vi "getMultiBarCode.vi"() -> ()   [LabVIEW 2012]
uses:
  <vilib>/vision/NI_Vision_Development_Module.lvlib
panel:
  out "String 4":string
  out "String 3":string
  out "String 2":string
  out "String":string
  in  "Stop":bool
  in  "Delay (s.)":dbl(slide)=0.4897959183673469 scale=0.0..2.0
  out "Code Read":string
  out "Image":T1(plugin-control)
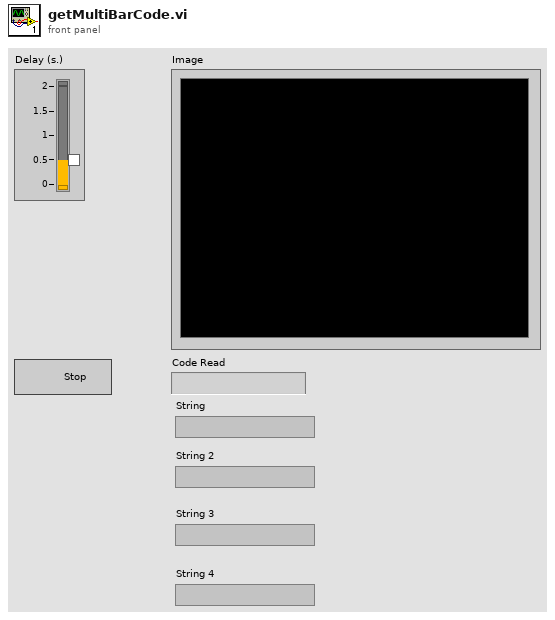
[diagram p1: front panel]
types:
  T1 = typedef "IMAQ Image.ctl" = refnum<image>
  T2 = typedef "IMAQ Rectangle" = cluster{"Left":i32, "Top":i32, "Right":i32, "Bottom":i32, "Rotation":dbl}
  T3 = typedef "ROI Descriptor" = cluster{"Global Rectangle":i32[], "Contours":cluster{"ID":enum32{"External", "Internal"}, "Type":u32, "Coordinates":i32[]}[]}
  T4 = cluster{"Special Char 1":string, "Special Char 2":string, "Confidence Level":sgl, "Barcode Type":u32}
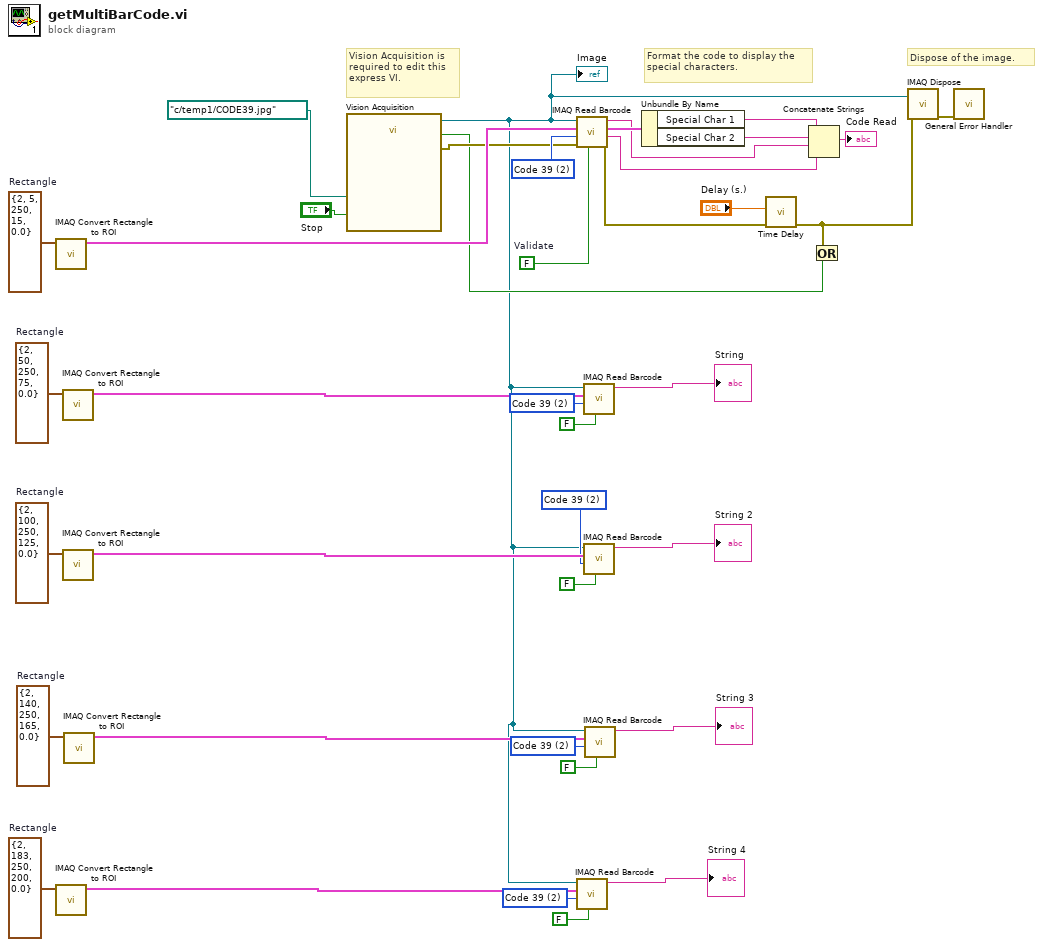
[diagram p0: block diagram]
diagram:
  w4 = u32 2 items=["Reserved", "Codabar", "Code 39", "Code 93", "Code 128", "EAN 8", "EAN 13", "Interleaved 2 of 5", "MSI", "UPCA", "Pharmacode", "RSS Limited"] ("Barcode Type")
  w6 = T2 {"Left"=2, "Top"=183, "Right"=250, "Bottom"=200, "Rotation"=0.0}  # Rectangle
  w9 = u32 2 items=["Reserved", "Codabar", "Code 39", "Code 93", "Code 128", "EAN 8", "EAN 13", "Interleaved 2 of 5", "MSI", "UPCA", "Pharmacode", "RSS Limited"] ("Barcode Type")
  w11 = T2 {"Left"=2, "Top"=140, "Right"=250, "Bottom"=165, "Rotation"=0.0}  # Rectangle
  w14 = u32 2 items=["Reserved", "Codabar", "Code 39", "Code 93", "Code 128", "EAN 8", "EAN 13", "Interleaved 2 of 5", "MSI", "UPCA", "Pharmacode", "RSS Limited"] ("Barcode Type")
  w16 = T2 {"Left"=2, "Top"=100, "Right"=250, "Bottom"=125, "Rotation"=0.0}  # Rectangle
  w19 = u32 2 items=["Reserved", "Codabar", "Code 39", "Code 93", "Code 128", "EAN 8", "EAN 13", "Interleaved 2 of 5", "MSI", "UPCA", "Pharmacode", "RSS Limited"] ("Barcode Type")
  w21 = T2 {"Left"=2, "Top"=50, "Right"=250, "Bottom"=75, "Rotation"=0.0}  # Rectangle
  w22 = FALSE  # Validate
  w35 = u32 2 items=["Reserved", "Codabar", "Code 39", "Code 93", "Code 128", "EAN 8", "EAN 13", "Interleaved 2 of 5", "MSI", "UPCA"] ("Barcode Type")
  w37 = T2 {"Left"=2, "Top"=5, "Right"=250, "Bottom"=15, "Rotation"=0.0}  # Rectangle
  # "Vision Acquisition is required to edit this express VI."
  # "Format the code to display the special characters."
  # "Dispose of the image."
  n1 = call "IMAQ Convert Rectangle to ROI"("Rectangle"=w37) -> ("ROI Descriptor"=w36:T3)  [unwired: 8 in, 1 out]
  n2 = call "IMAQ Convert Rectangle to ROI"("Rectangle"=w6) -> ("ROI Descriptor"=w5:T3)  [unwired: 8 in, 1 out]
  n3 = call "IMAQ Convert Rectangle to ROI"("Rectangle"=w21) -> ("ROI Descriptor"=w20:T3)  [unwired: 8 in, 1 out]
  n4 = call "IMAQ Convert Rectangle to ROI"("Rectangle"=w16) -> ("ROI Descriptor"=w15:T3)  [unwired: 8 in, 1 out]
  n5 = call "IMAQ Convert Rectangle to ROI"("Rectangle"=w11) -> ("ROI Descriptor"=w10:T3)  [unwired: 8 in, 1 out]
  n6 = call "Vision Acquisition"("Image Path"=path "c:/temp1/CODE39.jpg", "Stop (F)"="Stop") -> ("Image Out"=w1:T1, "Stopped"=w25:bool, "error out"=w26:errorcluster)  [unwired: 23 in]
  "Image" <- w1
  n7 = call "IMAQ Read Barcode"("Validate"=w22, "error in (no error)"=w26, "Barcode Type"=w35, "ROI Descriptor"=w36, "Image"=w1) -> ("error out"=w28:errorcluster, "Checksum(s)"=w29:string, "Extra Info"=w34:T4, "String"=w31:string)  [unwired: 3 out]
  n8 = call "IMAQ Read Barcode"("Validate"=FALSE, "Barcode Type"=w4, "ROI Descriptor"=w5, "Image"=w1) -> ("String"=→"String 4":string)  [unwired: 1 in, 6 out]
  n9 = call "IMAQ Read Barcode"("Validate"=FALSE, "Barcode Type"=w19, "ROI Descriptor"=w20, "Image"=w1) -> ("String"=→"String":string)  [unwired: 1 in, 6 out]
  n10 = call "IMAQ Read Barcode"("Validate"=FALSE, "Barcode Type"=w14, "ROI Descriptor"=w15, "Image"=w1) -> ("String"=→"String 2":string)  [unwired: 1 in, 6 out]
  n11 = call "IMAQ Read Barcode"("Validate"=FALSE, "Barcode Type"=w9, "ROI Descriptor"=w10, "Image"=w1) -> ("String"=→"String 3":string)  [unwired: 1 in, 6 out]
  n12 = Unbundle By Name(w34) -> ("Special Char 1"=w33:string, "Special Char 2"=w32:string)
  n13 = call "Time Delay"("error in (no error)"=w28, "Delay Time (s)"="Delay (s.)") -> ("error out"=w39:errorcluster)  [unwired: 9 in]
  n14 = Concatenate Strings(w33, w32, w31, w29) -> (→"Code Read":string)
  n15 = Or(x=w39, y=w25) -> ()  [unwired: 1 out]
  n16 = call "IMAQ Dispose"("Image"=w1, "error in (no error)"=w39) -> ("error out"=w38:errorcluster)  [unwired: 1 in, 3 out]
  n17 = call <vilib>:"General Error Handler.vi"("error in (no error)"=w38) -> ()  [unwired: 10 in, 5 out]
